vi "Read Measurement Times.vi"(8 "error in (no error)":errorcluster, 11 "SPECAN_PVT In":refnum<class "SPECAN_PVT.lvclass">) -> (0 "error out":errorcluster, 2 "Measurement Times":string[](array[string]), 3 "SPECAN_PVT Out":refnum<class "SPECAN_PVT.lvclass">)   [LabVIEW 2018, in "SPECAN_PVT.lvlib" / "SPECAN_PVT.lvclass"]
uses:
  SPECAN_PVT.lvclass
  SPECAN_PVT.lvclass/SPECAN_PVT.ctl
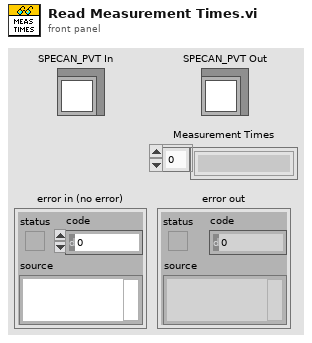
[diagram p1: front panel]
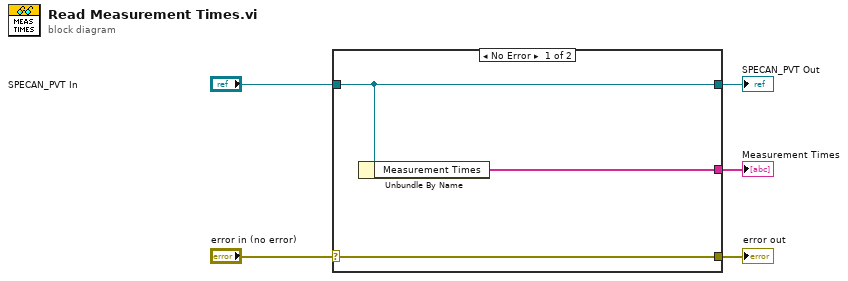
[diagram p0: block diagram]
diagram:
  n1 = case shown="No Error" "error in (no error)" {
    selector: "error in (no error)" -> [w8 w9]
    tunnel: [w8 w9] -> w4
    tunnel: [w7 w10] -> w2
    tunnel: "SPECAN_PVT In" -> [w7 w10]
    tunnel: [w6 _] -> w1
    frame No Error {
      n2 = Unbundle By Name(w7) -> ("Measurement Times"=w6:string[])
    }
    frame Error {
    }
  }
  "error out" <- w4
  "SPECAN_PVT Out" <- w2
  "Measurement Times" <- w1
